vi "fgt init Ex.vi"(8 "error in (no error)":errorcluster, 11 "SN":u16[](array[numeric])=array[4097 elements]) -> (0 "error out":errorcluster, 3 "SN out":u16[](array[numeric]))   [LabVIEW 2016, in "fgt_SDK.lvlib"]
doc: "Initialize specific Fluigent instrument(s) from their unique serial number. This function can be used when multiple instruments are connected in order to select your device(s)"
uses:
  fgt_SDK.lvlib
  dlls/fgt_SDK_32.dll
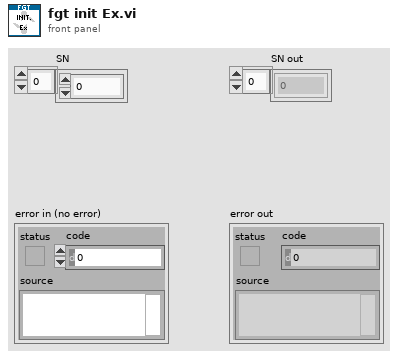
[diagram p1: front panel]
types:
  T1 = typedef "fgt_SDK.lvlib/fgt_STATUS_INFO.ctl" = cluster{"InstrType":T2, "instrSN":u16, "errorCode":u8, "infoCode":u8, "detail":string}
  T2 = typedef "fgt_SDK.lvlib/fgt_INSTRUMENT_TYPE.ctl" = enum32{"None", "MFCS", "MFCS_EZ", "FRP", "LineUP", "IPS"}
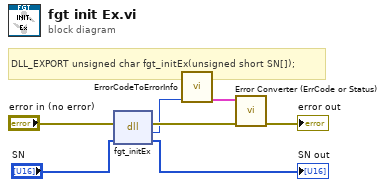
[diagram p0: block diagram]
diagram:
  # "DLL_EXPORT unsigned char fgt_initEx(unsigned short SN[]);"
  n1 = dll-call lib="C:/projects/SDK/fgt-sdk-labview/dlls/fgt_SDK_*.*" fn="fgt_initEx"(error in="error in (no error)", "SN"="SN") -> (error out=w4:errorcluster, "return type"=w2:u8, "SN"=→"SN out":u16[])  [unwired: 2 in, 1 out]
  n2 = call "ErrorCodeToErrorInfo.vi"("return type"=w2) -> ("StatusInfo"=w1:T1)  [unwired: 10 in]
  n3 = call "Error Converter (ErrCode or Status).vi"("error in (no error)"=w4, "StatusInfo"=w1) -> ("error out"=→"error out":errorcluster)  [unwired: 9 in]
